vi "my_3rd_vi_bis.vi"() -> ()   [LabVIEW 2019]
panel:
  out "Command":string
  in  "Input parameters":T1
  out "y white":i32[](array[numeric])
  out "x white":i32[](array[numeric])
  out "y yellow":i32[](array[numeric])
  out "x yellow":i32[](array[numeric])
  out "y red":i32[](array[numeric])
  out "x red":i32[](array[numeric])
  out "pos":string
  out "error out":errorcluster
  out "standard error":string
  out "standard output":string
  in  "error in (no error)":errorcluster
  out "Pixmap":u32[](array[numeric])
  out "hauteur":i16
  out "largeur":i16
  out "image":u8[](array[numeric])
  out "image depth":i32
  out "PNG Picture":picture
  in  "Path":path
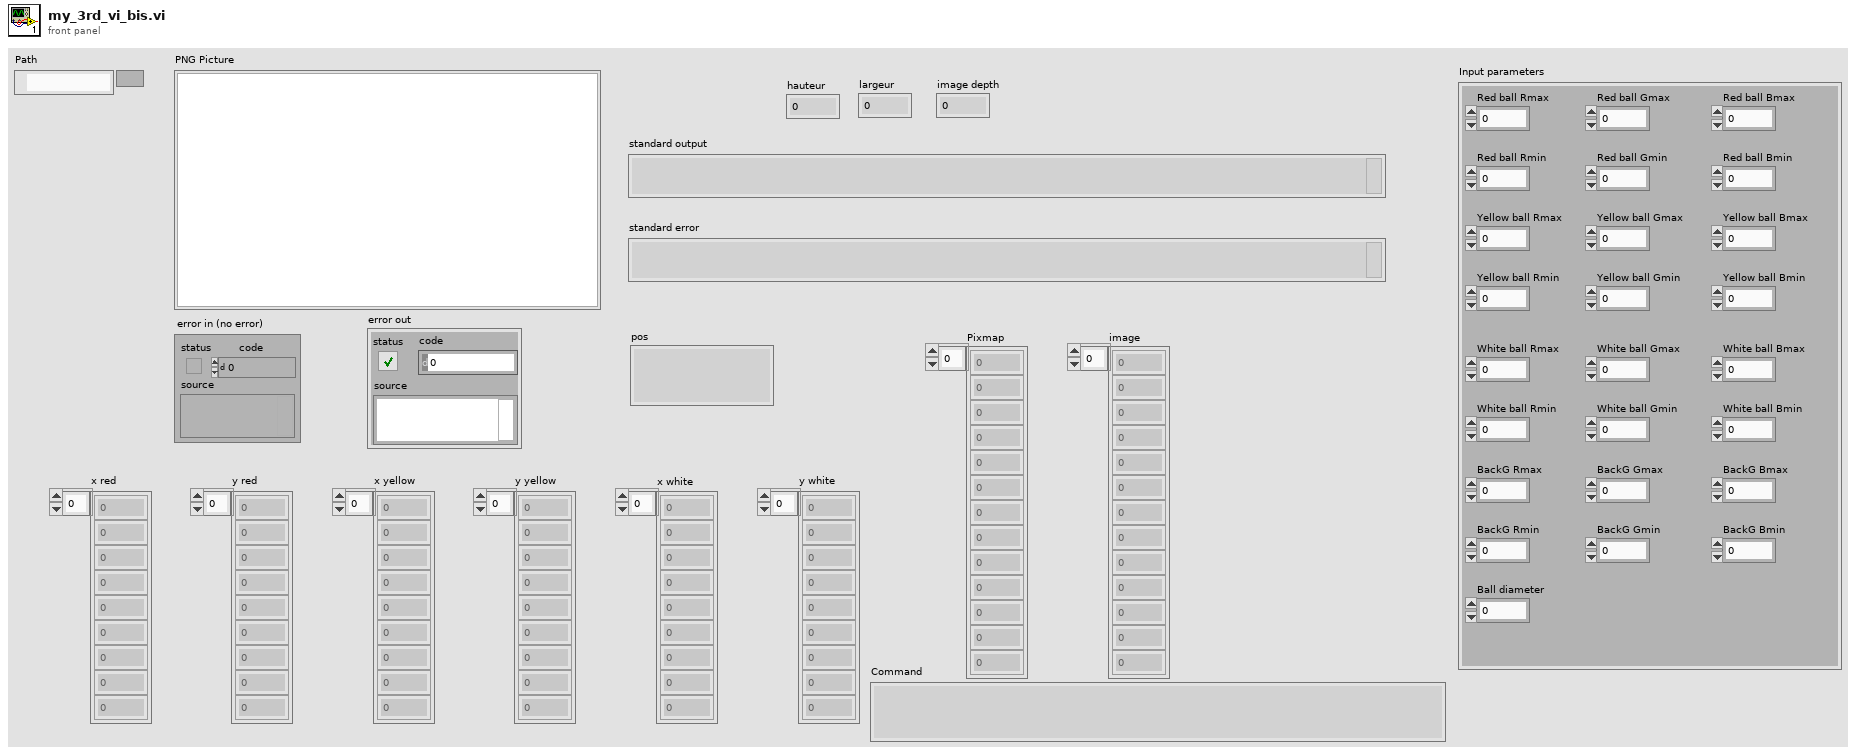
[diagram p1: front panel]
types:
  T1 = cluster{"Red ball Rmax":u8, "Red ball Gmax":u8, "Red ball Bmax":u8, "Red ball Rmin":u8, "Red ball Gmin":u8, "Red ball Bmin":u8, "Yellow ball Rmax":u8, "Yellow ball Gmax":u8, "Yellow ball Bmax":u8, "Yellow ball Rmin":u8, "Yellow ball Gmin":u8, "Yellow ball Bmin":u8, "White ball Rmax":u8, "White ball Gmax":u8, "White ball Bmax":u8, "White ball Rmin":u8, "White ball Gmin":u8, "White ball Bmin":u8, "BackG Rmax":u8, "BackG Gmax":u8, "BackG Bmax":u8, "BackG Rmin":u8, "BackG Gmin":u8, "BackG Bmin":u8, "Ball diameter":u8}
  T2 = cluster{"x red":i32, "y red":i32, "x yellow":i32, "y yellow":i32, "x white":i32, "y white":i32}
  T3 = enum16{"big-endian, network order", "native, host order", "little-endian"}
  T4 = typedef "imagedata.ctl" = cluster{"image type":i32, "image depth":i32, "image":u8[], "mask":u8[], "colors":u32[], "Rectangle":cluster{"left":i16, "top":i16, "right":i16, "bottom":i16}}
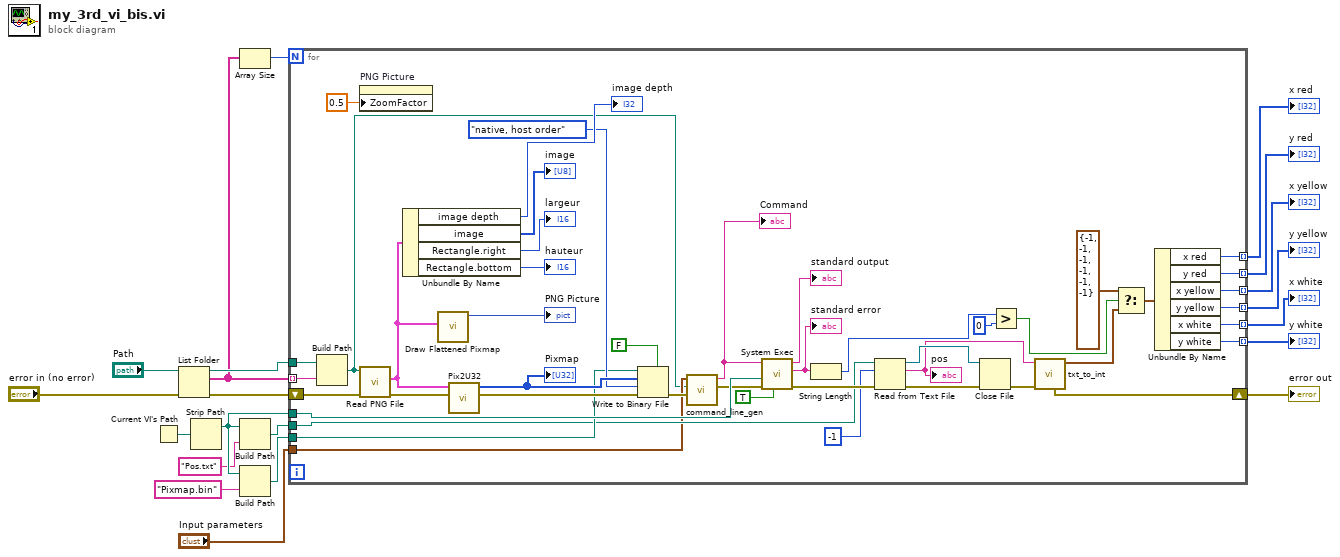
[diagram p0: block diagram]
diagram:
  n1 = Current VI's Path() -> (path=w15:path)
  n2 = List Folder(path="Path", error in="error in (no error)") -> (path out=w18:path, filenames=w9:string[], error out=w16:errorcluster)  [unwired: 2 in, 1 out]
  n3 = Strip Path(path=w15) -> (stripped path=w14:path)  [unwired: 1 out]
  n4 = Array Size(array=w9) -> (size(s)=w8:i32)
  n5 = Build Path(base path=w14, name or relative path="Pos.txt") -> (appended path=w10:path)
  n6 = Build Path(base path=w14, name or relative path="Pixmap.bin") -> (appended path=w12:path)
  n7 = for {
    N: w8 -> [_]
    tunnel: w18 -> [w46]
    tunnel: w9 -> [w45] mode=indexing
    tunnel: w14 -> [w44]
    tunnel: w12 -> [w43]
    tunnel: w10 -> [w42]
    tunnel: [w38] -> w7 mode=indexing
    tunnel: [w37] -> w6 mode=indexing
    tunnel: [w36] -> w5 mode=indexing
    tunnel: [w35] -> w4 mode=indexing
    tunnel: [w34] -> w3 mode=indexing
    tunnel: [w33] -> w2 mode=indexing
    shift-right: [w39] -> w20
    shift-left: w16 -> [w47]
    tunnel: "Input parameters" -> [w23]
    n8 = Build Path(base path=w46, name or relative path=w45) -> (appended path=w22:path)
    n9 = property on="PNG Picture" class="Pict"("ZoomFactor"=sgl 0.5 ("Zoom Factor")) -> ()  [unwired: 2 in, 2 out]
    n10 = call <vilib>:"Read PNG File.vi"("error in (no error)"=w47, "path to PNG file"=w22) -> ("error out"=w60:errorcluster, "image data"=w55:T4)  [unwired: 7 in, 1 out]
    n11 = Unbundle By Name(w55) -> ("image depth"=→"image depth":i32, "image"=→"image":u8[], "Rectangle.right"=→"largeur":i16, "Rectangle.bottom"=→"hauteur":i16)
    n12 = call <vilib>:"Draw Flattened Pixmap.vi"("image data"=w55) -> ("new picture"=→"PNG Picture":picture)  [unwired: 8 in]
    n13 = call "Pix2U32.vi"("error in (no error)"=w60, "input cluster"=w55) -> ("error out"=w61:errorcluster, "appended array"=w59:u32[])  [unwired: 8 in]
    "Pixmap" <- w59
    n14 = Write to Binary File(file (use dialog)=w43, data=w59, error in=w61, 5:FALSE ("prepend array or string size? (T)"), 9:T3."native, host order" ("byte order (0:big-endian, network order)")) -> (error out=w25:errorcluster)  [unwired: 1 in, 2 out]
    n15 = call "command_line_gen.vi"("error in (no error)"=w25, "Path"=w22, "Input parameters"=w23) -> ("error out"=w24:errorcluster, "Command"=w21:string)  [unwired: 7 in]
    "Command" <- w21
    n16 = call <vilib>:"System Exec.vi"("run minimized? (F)"=TRUE, "error in (no error)"=w24, "working directory"=w44, "command line"=w21) -> ("error out"=w65:errorcluster, "standard error"=w26:string, "standard output"=→"standard output":string)  [unwired: 4 in, 1 out]
    "standard error" <- w26
    n17 = String Length(string=w26) -> (length=w29:i32)
    n18 = Read from Text File(file (use dialog)=w42, count=-1, error in=w65) -> (refnum out=w63:refnum<file>, text=w41:string, error out=w64:errorcluster)  [unwired: 1 in, 1 out]
    "pos" <- w41
    n19 = Close File(refnum=w63, error in=w64) -> (error out=w40:errorcluster)  [unwired: 1 out]
    n20 = Greater?(x=w29, y=0) -> (0:w27:bool)
    n21 = call "txt_to_int.vi"("error in (no error)"=w40, "pos.txt"=w41) -> ("Cluster"=w32:T2, "error out"=w39:errorcluster)  [unwired: 5 in, 3 out]
    n22 = Select(t=T2 {"x red"=-1, "y red"=-1, "x yellow"=-1, "y yellow"=-1, "x white"=-1, "y white"=-1}, s=w27, f=w32) -> (s? t:f=w31:T2)
    n23 = Unbundle By Name(w31) -> ("x red"=w38:i32, "y red"=w37:i32, "x yellow"=w36:i32, "y yellow"=w35:i32, "x white"=w34:i32, "y white"=w33:i32)
  }
  "error out" <- w20
  "x red" <- w7
  "y red" <- w6
  "x yellow" <- w5
  "y yellow" <- w4
  "x white" <- w3
  "y white" <- w2
